vi "_caraya_updateLibraryIcon.vi"(8 "error in (no error)":errorcluster, 10 "Application":refnum<vi>, 11 "Class Path":path=path "C:/Projects/JKI/Caraya/src/tests/test-all-asserts/Test Runner.AllAsserts.lvclass") -> (0 "error out":errorcluster)   [LabVIEW 2013]
uses:
  <vilib>/LabVIEW Icon API/API_Rectangle Dimension.ctl
  <vilib>/LabVIEW Icon API/API_Text.ctl
  <vilib>/LabVIEW Icon API/LabVIEW Icon API.lvlib
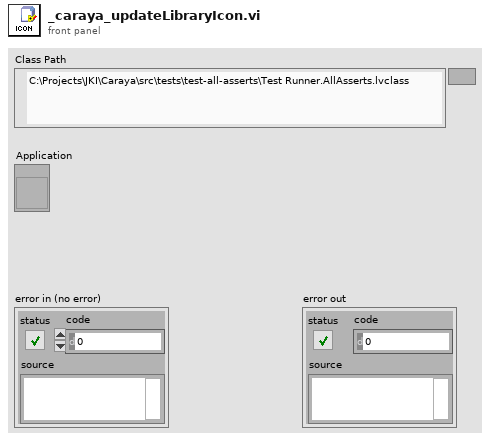
[diagram p1: front panel]
types:
  T1 = typedef "LabVIEW Icon API.lvlib/API_Text.ctl" = cluster{"Line 1 text":string, "Line 2 text":string, "Line 3 text":string, "Line 4 text":string}
  T2 = typedef "LabVIEW Icon API.lvlib/API_Rectangle Dimension.ctl" = cluster{"Width":i16, "Height":i16}
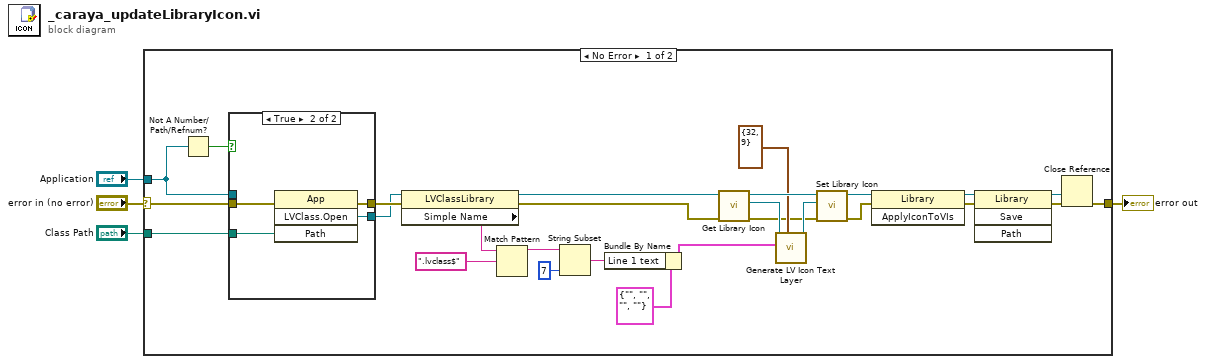
[diagram p0: block diagram]
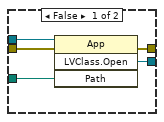
[diagram p2: hidden frame]
diagram:
  n1 = case shown="No Error" "error in (no error)" {
    selector: "error in (no error)" -> [w5 w41]
    tunnel: "Class Path" -> [w27 _]
    tunnel: [w26 w41] -> w3
    tunnel: "Application" -> [w25 _]
    frame No Error {
      n2 = Not A Number/Path/Refnum?(number/path/refnum=w25) -> (NaN/Path/Refnum?=w24:bool)
      n3 = case shown="True" w24 {
        tunnel: [w36 w40] -> w29
        tunnel: [w35 w39] -> w28
        tunnel: w27 -> [w34 w38]
        tunnel: w5 -> [w33 w37]
        tunnel: w25 -> [w32 _]
        frame False {
          n4 = invoke class="App" method="LVClass.Open"(reference=w32, error in=w33, "Path"=w34) -> (error out=w36:errorcluster, "LVClass.Open"=w35:refnum<vi>)  [unwired: 1 in, 2 out]
        }
        frame True {
          n5 = invoke class="App" method="LVClass.Open"(error in=w37, "Path"=w38) -> (error out=w40:errorcluster, "LVClass.Open"=w39:refnum<vi>)  [unwired: 2 in, 2 out]
        }
      }
      n6 = property class="LVClassLibrary"(reference=w28, error in=w29) -> (reference out=w14:refnum<vi>, error out=w8:errorcluster, "Simple Name"=w22:string)
      n7 = Match Pattern(string=w22, regular expression=".lvclass$") -> (before substring=w21:string)  [unwired: 1 in, 3 out]
      n8 = String Subset(string=w21, length (rest)=7 ("length (rest)")) -> (substring=w9:string)  [unwired: 1 in]
      n9 = Bundle By Name(cluster=T1 {"Line 1 text"="", "Line 2 text"="", "Line 3 text"="", "Line 4 text"=""} ("Text"), "Line 1 text"=w9) -> (w10:T1)
      n10 = call <vilib>:"Get Library Icon.vi"("error in (no error)"=w8, "Library Refnum in"=w14) -> ("error out"=w7:errorcluster, "Icon"=w16:refnum<class "Icon.lvclass">, "Library Refnum out"=w17:refnum<vi>)  [unwired: 7 in]
      n11 = call <vilib>:"Generate LV Icon Text Layer.vi"("Rectangle dimension (32,32)"=T2 {"Width"=32, "Height"=9}, "Text"=w10, "Icon in"=w16) -> ("Icon out"=w15:refnum<class "Icon.lvclass">)  [unwired: 7 in, 1 out]
      n12 = call <vilib>:"Set Library Icon.vi"("error in (no error)"=w7, "Icon"=w15, "Library Refnum in"=w17) -> ("error out"=w6:errorcluster, "Library Refnum out"=w13:refnum<vi>)  [unwired: 7 in]
      n13 = invoke class="Library" method="ApplyIconToVIs"(reference=w13, error in=w6) -> (reference out=w18:refnum<vi>, error out=w19:errorcluster)  [unwired: 1 in, 1 out]
      n14 = invoke class="Library" method="Save"(reference=w18, error in=w19) -> (reference out=w30:refnum<vi>, error out=w31:errorcluster)  [unwired: 2 in, 2 out]
      n15 = Close Reference(reference=w30, error in (no error)=w31) -> (error out=w26:errorcluster)
    }
    frame Error {
    }
  }
  "error out" <- w3
